vi "Result.Measurement Status to String.vi"(1 "Status":T1 items=["LOG", "PASS", "FAIL", "ERROR"]) -> (0 "resulting string":string)   [LabVIEW 2018]
uses:
  Result.Measurement and Attribute Item Status.ctl
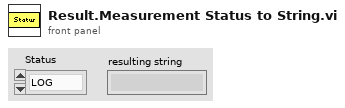
[diagram p1: front panel]
types:
  T1 = typedef "Result.Measurement and Attribute Item Status.ctl" = i32
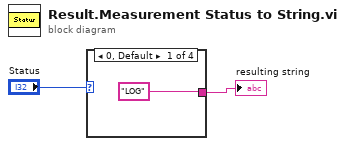
[diagram p0: block diagram]
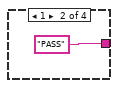
[diagram p2: hidden frame]
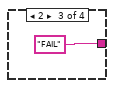
[diagram p3: hidden frame]
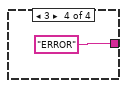
[diagram p4: hidden frame]
diagram:
  n1 = case shown="0, Default" "Status" {
    tunnel: ["LOG" "PASS" "FAIL" "ERROR"] -> w1
    frame 0, Default {
    }
    frame 1 {
    }
    frame 2 {
    }
    frame 3 {
    }
  }
  "resulting string" <- w1
